vi "Calc2.vi"() -> ()   [LabVIEW 2021]
panel:
  out "Numeric 2":dbl
  out "Numeric":dbl=695.0
  out "Operation":string
  in  "?":bool
  in  "?":bool
  in  "?":bool
  in  "?":bool
  in  "?":bool
  in  "?":bool
  in  "?":bool
  in  "?":bool
  in  "?":bool
  in  "?":bool
  in  "?":bool
  in  "?":bool
  in  "?":bool
  in  "?":bool
  in  "Equals":bool
  out "Output":dbl
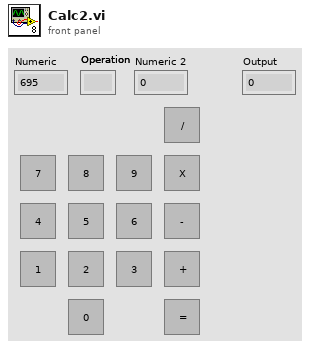
[diagram p1: front panel]
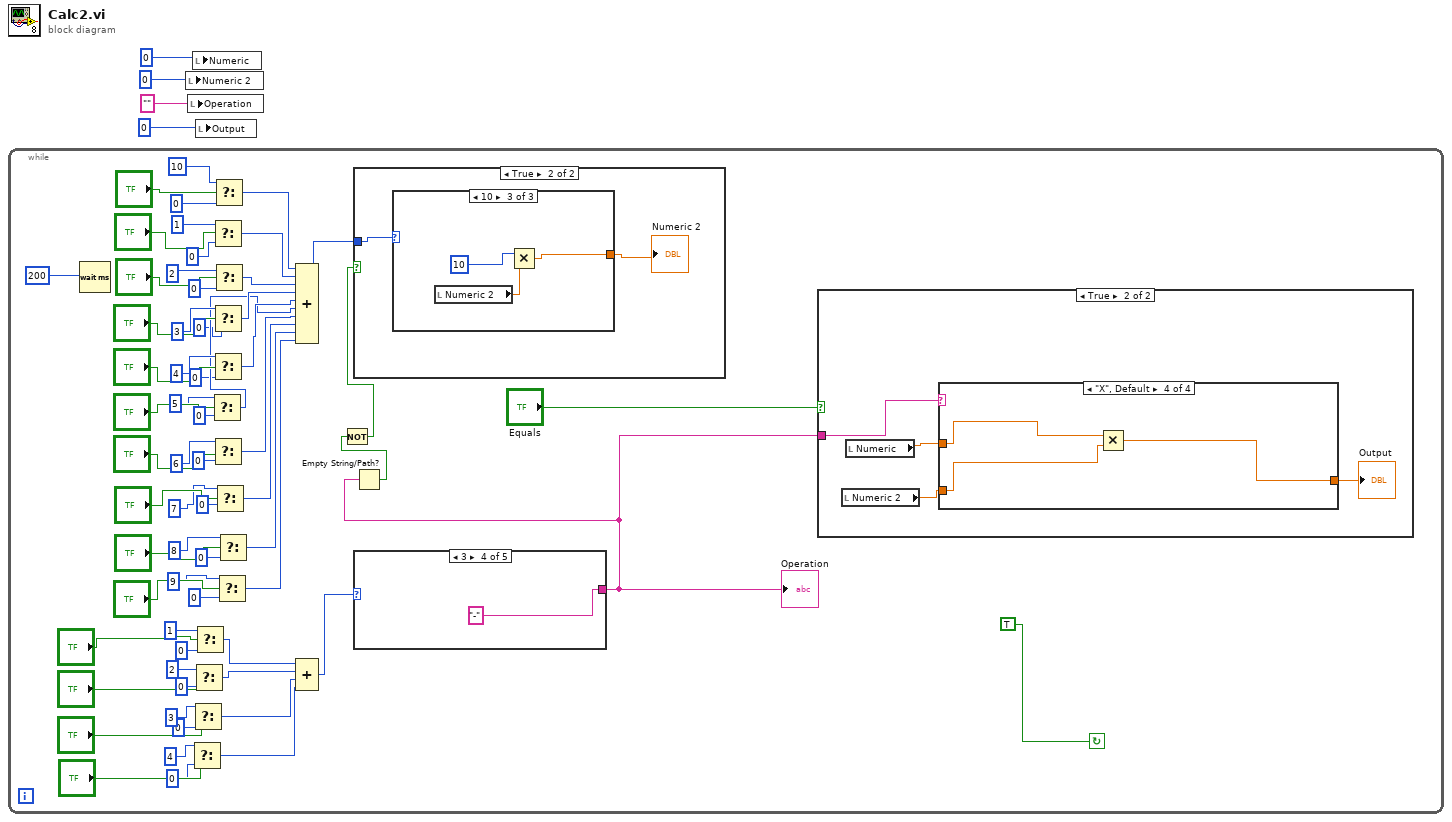
[diagram p0: block diagram]
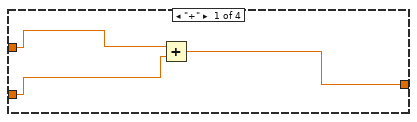
[diagram p3: hidden frame]
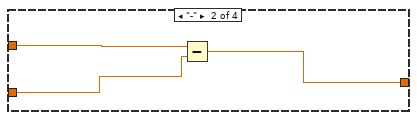
[diagram p4: hidden frame]
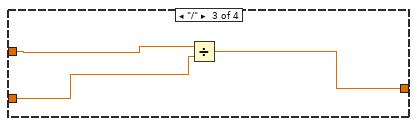
[diagram p5: hidden frame]
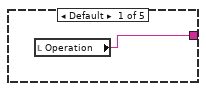
[diagram p6: hidden frame]
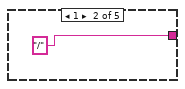
[diagram p7: hidden frame]
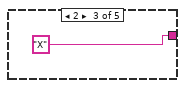
[diagram p8: hidden frame]
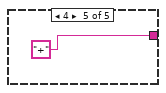
[diagram p9: hidden frame]
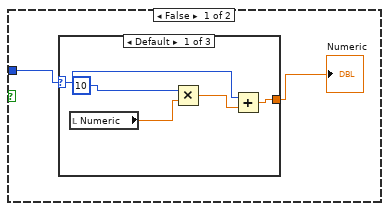
[diagram p10: hidden frame]
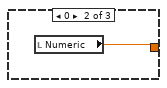
[diagram p11: hidden frame]
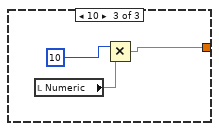
[diagram p12: hidden frame]
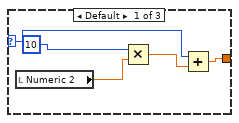
[diagram p13: hidden frame]
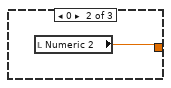
[diagram p14: hidden frame]
diagram:
  n1 = while {
    stop <- TRUE continue-if-true
    n2 = Wait (ms)(milliseconds to wait=200) -> ()  [unwired: 1 out]
    n3 = Select(t=4, s="?", f=0) -> (s? t:f=w26:i32)
    n4 = Select(t=3, s="?", f=0) -> (s? t:f=w27:i32)
    n5 = Select(t=2, s="?", f=0) -> (s? t:f=w28:i32)
    n6 = Select(t=1, s="?", f=0) -> (s? t:f=w29:i32)
    n7 = Select(t=5, s="?", f=0) -> (s? t:f=w43:i32)
    n8 = Select(t=1, s="?", f=0) -> (s? t:f=w47:i32)
    n9 = Select(t=3, s="?", f=0) -> (s? t:f=w45:i32)
    n10 = Select(t=4, s="?", f=0) -> (s? t:f=w44:i32)
    n11 = Select(t=6, s="?", f=0) -> (s? t:f=w42:i32)
    n12 = Select(t=10, s="?", f=0) -> (s? t:f=w48:i32)
    n13 = Select(t=2, s="?", f=0) -> (s? t:f=w46:i32)
    n14 = Select(t=7, s="?", f=0) -> (s? t:f=w41:i32)
    n15 = Select(t=9, s="?", f=0) -> (s? t:f=w39:i32)
    n16 = Select(t=8, s="?", f=0) -> (s? t:f=w40:i32)
    n17 = Compound Arithmetic op=ADD(w48, w47, w46, w45, w44, w43, w42, w41, w40, w39) -> (w38:i32)
    n18 = Compound Arithmetic op=ADD(w29, w28, w27, w26) -> (w10:i32)
    n19 = case shown="3" w10 {
      tunnel: [w85 "/" "X" "-" "+"] -> w8
      frame Default {
        n20 = local read "Operation"() -> (w85:string)
      }
      frame 1 {
      }
      frame 2 {
      }
      frame 3 {
      }
      frame 4 {
      }
    }
    "Operation" <- w8
    n21 = Empty String/Path?(string/path=w8) -> (empty?=w7:bool)
    n22 = Not(x=w7) -> (.not. x?=w6:bool)
    n23 = case shown="True" w6 {
      tunnel: w38 -> [w91 w102]
      frame False {
        n24 = case shown="Default" w91 {
          selector: w91 -> [w92 _ _]
          tunnel: [w93 w97 w98] -> w90
          frame Default {
            n25 = local read "Numeric"() -> (w96:dbl)
            n26 = Multiply(x=10, y=w96) -> (x*y=w94:dbl)
            n27 = Add(x=w92, y=w94) -> (x+y=w93:dbl)
          }
          frame 0 {
            n28 = local read "Numeric"() -> (w97:dbl)
          }
          frame 10 {
            n29 = local read "Numeric"() -> (w99:dbl)
            n30 = Multiply(x=10, y=w99) -> (x*y=w98:dbl)
          }
        }
        "Numeric" <- w90
      }
      frame True {
        n31 = case shown="10" w102 {
          selector: w102 -> [w103 _ _]
          tunnel: [w104 w108 w109] -> w101
          frame Default {
            n32 = local read "Numeric 2"() -> (w107:dbl)
            n33 = Multiply(x=10, y=w107) -> (x*y=w105:dbl)
            n34 = Add(x=w103, y=w105) -> (x+y=w104:dbl)
          }
          frame 0 {
            n35 = local read "Numeric 2"() -> (w108:dbl)
          }
          frame 10 {
            n36 = local read "Numeric 2"() -> (w110:dbl)
            n37 = Multiply(x=10, y=w110) -> (x*y=w109:dbl)
          }
        }
        "Numeric 2" <- w101
      }
    }
    n38 = case shown="True" "Equals" {
      tunnel: w8 -> [_ w69]
      frame False {
      }
      frame True {
        n39 = local read "Numeric 2"() -> (w70:dbl)
        n40 = local read "Numeric"() -> (w71:dbl)
        n41 = case shown="\"X\", Default" w69 {
          tunnel: w71 -> [w75 w78 w81 w84]
          tunnel: w70 -> [w74 w77 w80 w83]
          tunnel: [w73 w76 w79 w82] -> w72
          frame "+" {
            n42 = Add(x=w75, y=w74) -> (x+y=w73:dbl)
          }
          frame "-" {
            n43 = Subtract(x=w78, y=w77) -> (x-y=w76:dbl)
          }
          frame "/" {
            n44 = Divide(x=w81, y=w80) -> (x/y=w79:dbl)
          }
          frame "X", Default {
            n45 = Multiply(x=w84, y=w83) -> (x*y=w82:dbl)
          }
        }
        "Output" <- w72
      }
    }
  }
  n46 = local write "Numeric 2"(0) -> ()
  n47 = local write "Operation"("") -> ()
  n48 = local write "Numeric"(0) -> ()
  n49 = local write "Output"(0) -> ()
